vi "HandleCollectorWrap.vi"(7 "InitState":T1, 8 "error in (no error)":errorcluster, 11 "Toggle?":bool) -> (0 "error out":errorcluster, 2 "State":T1)   [LabVIEW 2013]
uses:
  CollectorWrapAction.ctl
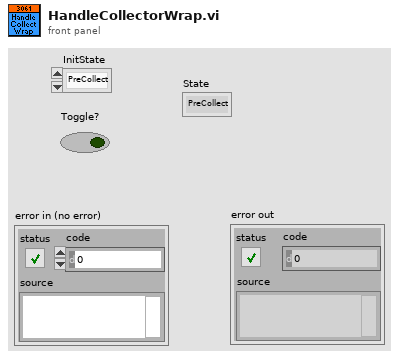
[diagram p1: front panel]
types:
  T1 = typedef "CollectorWrapAction.ctl" = enum16{"PreCollect", "Collect", "Stop"}
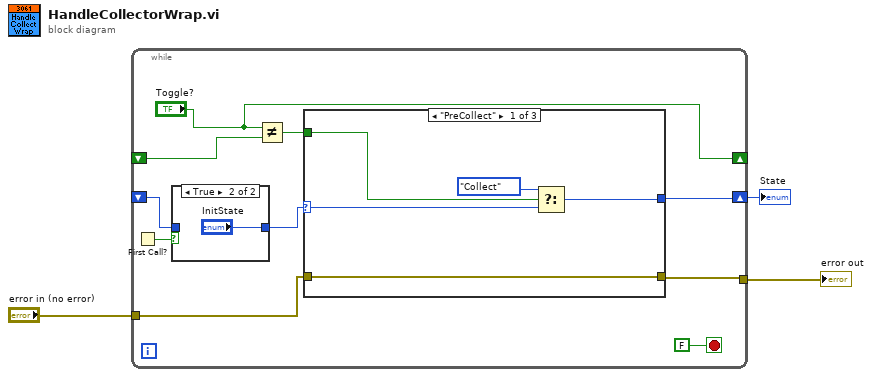
[diagram p0: block diagram]
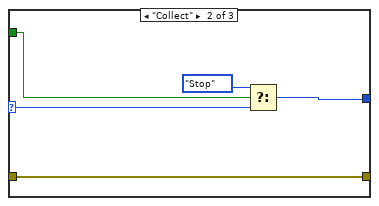
[diagram p3: hidden frame]
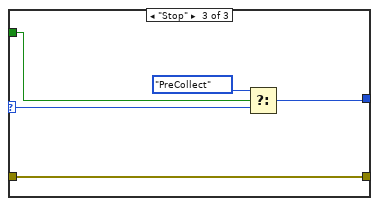
[diagram p4: hidden frame]
diagram:
  n1 = while {
    shift-right: [w7] -> w1
    shift-left: _ -> [w11]
    shift-right: ["Toggle?"] -> _
    shift-left: _ -> [w6]
    tunnel: "error in (no error)" -> [w10]
    tunnel: [w9] -> w2
    stop <- FALSE stop-if-true
    n2 = First Call?() -> (First Call?: T/F=w12:bool)
    n3 = case shown="True" w12 {
      tunnel: w11 -> [w14 _]
      tunnel: [w14 "InitState"] -> w8
      frame False {
      }
      frame True {
      }
    }
    n4 = Not Equal?(x="Toggle?", y=w6) -> (x != y?=w5:bool)
    n5 = case shown="\"PreCollect\"" w8 {
      selector: w8 -> [w20 w25 w30]
      tunnel: w10 -> [w17 w24 w26]
      tunnel: [w17 w24 w26] -> w9
      tunnel: [w19 w23 w27] -> w7
      tunnel: w5 -> [w16 w22 w29]
      frame "PreCollect" {
        n6 = Select(t=CollectorWrapAction."Collect", s=w16, f=w20) -> (s? t:f=w19:T1)
      }
      frame "Collect" {
        n7 = Select(t=CollectorWrapAction."Stop", s=w22, f=w25) -> (s? t:f=w23:T1)
      }
      frame "Stop" {
        n8 = Select(t=CollectorWrapAction."PreCollect", s=w29, f=w30) -> (s? t:f=w27:T1)
      }
    }
  }
  "error out" <- w2
  "State" <- w1
